vi "Write Attribute Pointer Flag.vi"(10 "Attribute Pointer?":bool[](array[boolean]), 11 "Test Step Dialog in":refnum<class "Test Step Dialog.lvclass">) -> (3 "Test Step Dialog out":refnum<class "Test Step Dialog.lvclass">)   [LabVIEW 2017, in "Test Step Dialog.lvclass"]
uses:
  <vilib>/gpm_packages/@cs/Test-executive-builder/Source/Test Executive Builder Dialogs/Test Step Dialog/Test Step Dialog.lvclass
  <vilib>/gpm_packages/@cs/Test-executive-builder/Source/Test Executive Builder Dialogs/Test Step Dialog/Test Step Dialog.lvclass/Test Step Dialog.ctl
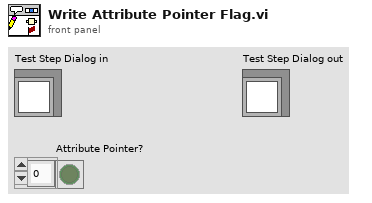
[diagram p1: front panel]
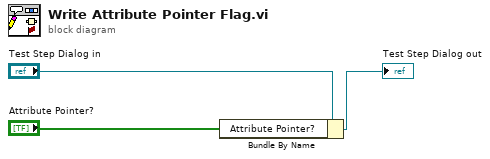
[diagram p0: block diagram]
diagram:
  n1 = Bundle By Name(cluster="Test Step Dialog in", "Attribute Pointer?"="Attribute Pointer?") -> (→"Test Step Dialog out":refnum<class "Test Step Dialog.lvclass">)
